vi "SeCrTs-Abort Executer.vi"(8 "error in":errorcluster, 11 "Message Queue":refnum<queue>) -> (0 "error IO":errorcluster)   [LabVIEW 2022 SP3]
uses:
  <vilib>/Platform/TimedLoop/XDataNode/timing_clust.ctl
  <vilib>/Platform/TimedLoop/XDataNode/nitl_modes.ctl
  <vilib>/Platform/TimedLoop/XDataNode/wakeup.ctl
  <vilib>/platform/TimedLoop/XDataNode/XDataNode.xnode
  <vilib>/Platform/TimedLoop/XDataNode/XDNodeRunTimeDep.lvlib
panel:
  out "Numeric":i32
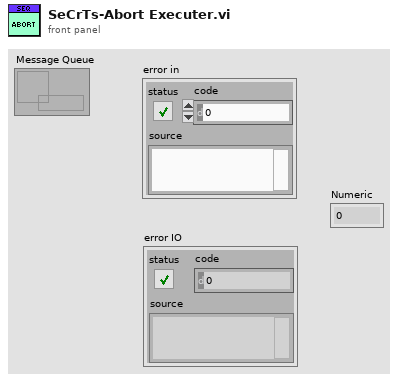
[diagram p1: front panel]
types:
  T1 = typedef "XDNodeRunTimeDep.lvlib/timing_clust.ctl" = cluster{"Expected End [f-1]":u64, "Actual End [f-1]":u64, "Finished Late? [f-1]":bool, "Expected End [i-1]":u64, "Actual End [i-1]":u64, "Finished Late? [i-1]":bool, "Expected Start [i]":u64, "Actual Start [i]":u64, "Expected Start [f]":u64, "Actual Start [f]":u64, "Source Name":string, "Structure Name":string, "Period":i64, "Deadline":i64, "Offset":i64, "Start":i64, "Priority":i32, "Timeout":i32, "Mode":T2, "Wakeup Reason":T3, "Error":errorcluster, "Source Type":string, "Secondary Source Type":string, "Global End Time":u64, "Global Start Time":u64, "Frame Duration":u64, "Iteration Duration":u64, "Assigned CPU":i32, "I/O Scan Engine Mode":u32}
  T2 = typedef "XDNodeRunTimeDep.lvlib/nitl_modes.ctl" = enum32{"No Change", "Process missed periods, maintain original phase", "Discard missed periods, maintain original phase", "Process missed periods, ignore original phase", "Discard missed periods, ignore original phase"}
  T3 = typedef "XDNodeRunTimeDep.lvlib/wakeup.ctl" = enum32{"Normal", "Aborted", "Asynchronous wakeup", "Timing source error", "Timed loop error", "Timeout"}
  T4 = enum16{"Init", "Read", "Write 'All'", "Write 'n'", "Write Safe Value", "Write Start Time", "Overwrite Pattern", "Overwrite Pattern with Start", "Append Pattern", "Start Pattern Mode", "Abort Pattern Mode", "Read 1"}
  T5 = cluster{"Start DAQ":bool, "Stop DAQ":bool, "RT Stop":bool, "RT Exit":bool, "Start Seq":bool}
  T6 = cluster{"Manual HOLD":bool, "Automatic Hold AI":bool, "Abort":bool, "Automatic Hold DI":bool}
  T7 = cluster{cluster{"Sr. No.":string, "Time CDT":string, "Component ID":string, "Data Type":string, "Condition":string, "Range/Position":string, "No of Samples for Pass":string, "Event Duration":string, "Continuous /Cumulative":string, "Expected Delay":string, "Failure case Seq":string, "Current Sequence":string}[]}[]
  T8 = cluster{"Sr. No.":string, "Time CDT":string, "Component ID":string, "Data Type":string, "Condition":string, "Range/Position":string, "No of Samples for Pass":string, "Event Duration":string, "Continuous /Cumulative":string, "Expected Delay":string, "Failure case Seq":string, "Current Sequence":string}[]
  T9 = cluster{"Sr. No.":string, "Time CDT":string, "Component ID":string, "Data Type":string, "Condition":string, "Range/Position":string, "No of Samples for Pass":string, "Event Duration":string, "Continuous /Cumulative":string, "Expected Delay":string, "Failure case Seq":string, "Current Sequence":string}
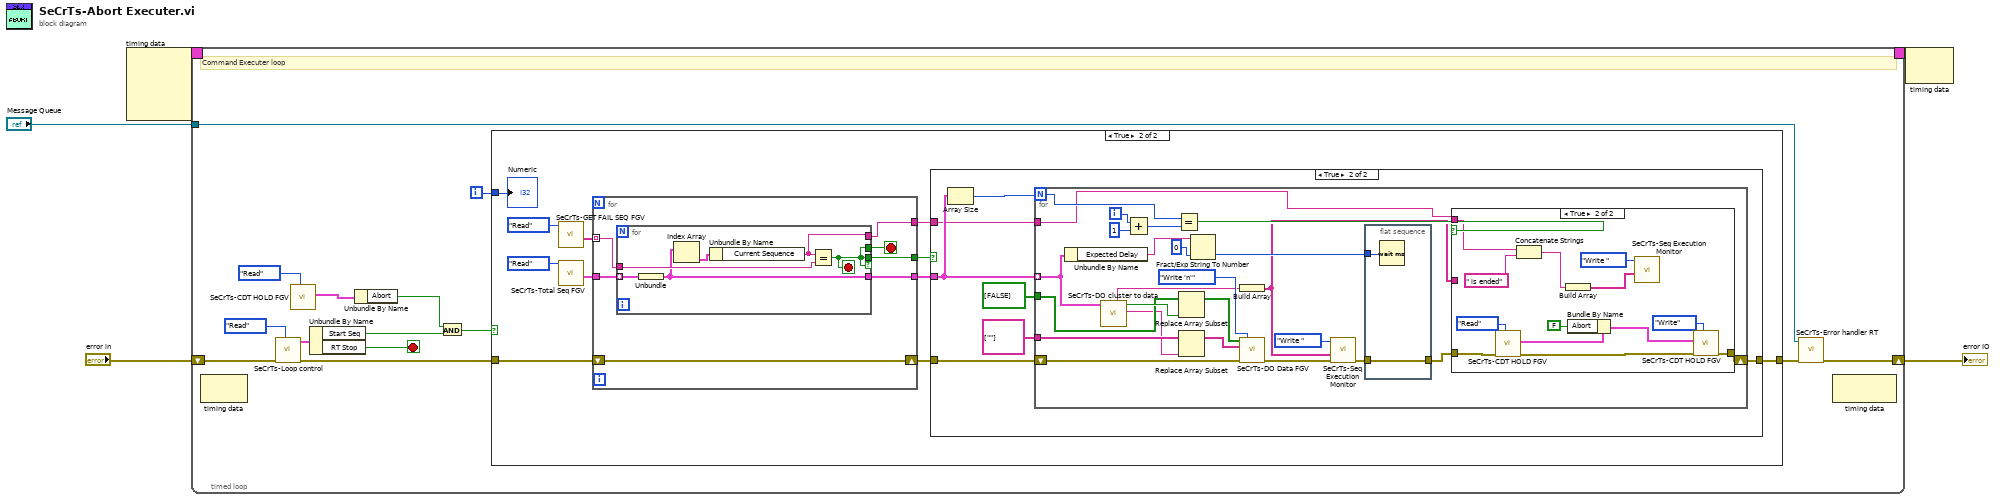
[diagram p0: block diagram]
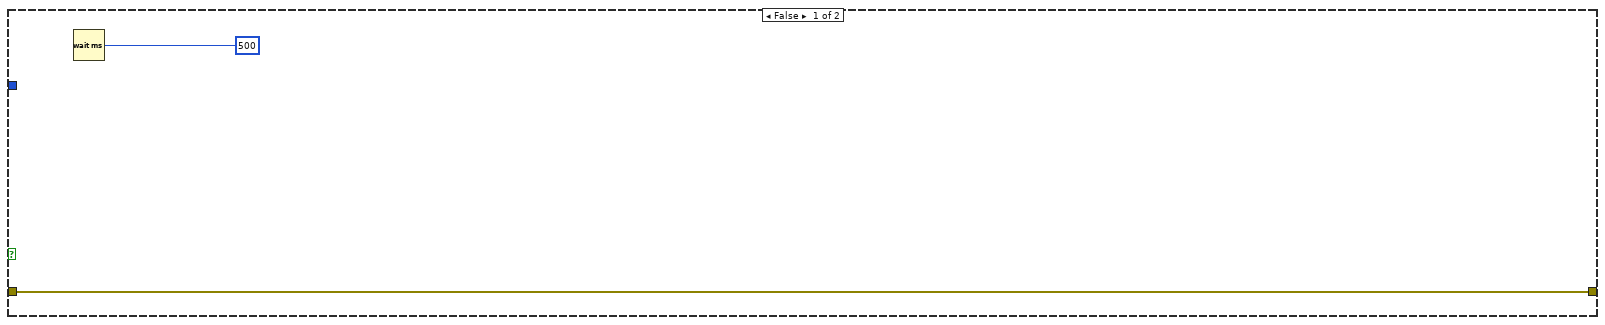
[diagram p2: hidden frame]
diagram:
  n1 = node-c288() -> (w3:T1)  [unwired: 4 in]
  n2 = timed-loop {
    shift-right: [w12] -> w4
    shift-left: "error in" -> [w17]
    timing: w3 -> [_]
    timing-out: [_] -> w2
    tunnel: "Message Queue" -> [w11]
    i -> [w18]
    stop <- w19 stop-if-true
    # "Command Executer loop"
    n3 = node-c288() -> ()  [unwired: 1 in, 1 out]
    n4 = call "SeCrTs-Loop control.vi"("Action"=enum16{"Init", "Write", "Read"}."Read", "error in (no error)"=w17) -> ("error Out"=w16:errorcluster, "Loop Control out"=w14:T5)  [unwired: 8 in]
    n5 = call "SeCrTs-CDT HOLD FGV.vi"("Write/Read"=enum16{"Write", "Read"}."Read") -> ("HOLD and Abort Out"=w8:T6)  [unwired: 7 in, 1 out]
    n6 = Unbundle By Name(w14) -> ("Start Seq"=w9:bool, "RT Stop"=w19:bool)
    n7 = Unbundle By Name(w8) -> ("Abort"=w6:bool)
    n8 = And(x=w6, y=w9) -> (x .and. y?=w7:bool)
    n9 = case shown="True" w7 {
      tunnel: [w21 w32] -> w13
      tunnel: w18 -> [_ w31]
      tunnel: w16 -> [w21 w24]
      frame False {
        n10 = Wait (ms)(milliseconds to wait=u32 500) -> ()  [unwired: 1 out]
      }
      frame True {
        n11 = call "SeCrTs-GET FAIL SEQ FGV.vi"("Enum"=enum16{"Read", "Write "}."Read") -> ("Failure \ncase Seq"=w25:string[])  [unwired: 9 in, 1 out]
        n12 = call "SeCrTs-Total Seq FGV.vi"("Enum"=enum16{"Read", "Write "}."Read") -> ("Total Seq  Out"=w28:T7)  [unwired: 9 in, 1 out]
        n13 = for {
          tunnel: [w35] -> w26
          tunnel: w28 -> [w36]
          tunnel: w25 -> [w39] mode=indexing
          tunnel: [w38] -> w27
          shift-right: [w34] -> w23
          shift-left: w24 -> [w34]
          tunnel: [w33] -> w22
          stop <- w37 stop-if-true
          n14 = for {
            tunnel: [w44] -> w38 if=w44
            tunnel: w39 -> [w45]
            tunnel: [w44] -> w37
            tunnel: w36 -> [w42] mode=indexing
            tunnel: [w41] -> w35
            tunnel: [w40] -> w33
            stop <- w44 stop-if-true
            n15 = Unbundle(w42) -> (w41:T8)
            n16 = Index Array(array=w41) -> (element=w43:T9)  [unwired: 1 in]
            n17 = Unbundle By Name(w43) -> ("Current Sequence"=w40:string)
            n18 = Equal?(x=w40, y=w45) -> (x = y?=w44:bool)
          }
        }
        n19 = case shown="True" w27 {
          tunnel: w23 -> [w46 w50]
          tunnel: [w46 w53] -> w32
          tunnel: w26 -> [_ w49]
          tunnel: w22 -> [_ w47]
          frame False {
          }
          frame True {
            n20 = Array Size(array=w49) -> (size(s)=w48:i32)
            n21 = for {
              N: w48 -> [w59]
              tunnel: w49 -> [w70] mode=indexing
              tunnel: string[] [""] ("appended array") -> [w78]
              tunnel: bool[] [FALSE] ("appended array") -> [w76]
              shift-right: [w56] -> w53
              shift-left: w50 -> [w71]
              tunnel: w47 -> [w55]
              i -> [w62]
              n22 = Unbundle By Name(w70) -> ("Expected Delay"=w73:string)
              n23 = call "SeCrTs-DO cluster to data.vi"("output cluster"=w70) -> ("Component ID"=w66:string, "Boolean"=w77:bool, "Sequence"=w63:string)  [unwired: 7 in, 1 out]
              n24 = Add(x=w62, y=1) -> (x+y=w60:i32)
              n25 = Equal?(x=w59, y=w60) -> (x = y?=w58:bool)
              n26 = Replace Array Subset(array=w76, new element=w77) -> (w75:bool[])  [unwired: 1 in]
              n27 = Replace Array Subset(array=w78, new element=w66) -> (w74:string[])  [unwired: 1 in]
              n28 = Fract/Exp String To Number(string=w73, default (0 dbl)=u32 0 ("y")) -> (number=w68:u32)  [unwired: 2 in, 1 out]
              n29 = Build Array(w63) -> (w54:string[])
              n30 = call "SeCrTs-DO Data FGV.vi"("DO Values In"=w75, "Option"=T4."Write 'n'", "DO Channel Names"=w74, "error in (no error)"=w71) -> ("error out"=w65:errorcluster)  [unwired: 5 in, 6 out]
              n31 = call "SeCrTs-Seq Execution Monitor.vi"("error in"=w65, "Seq Monitor"=w54, "Enum"=enum16{"Read", "Write "}."Write ") -> ("error out"=w64:errorcluster)  [unwired: 7 in, 1 out]
              n32 = flat-sequence {
                tunnel: w64 -> [w94]
                tunnel: [w94] -> w57
                tunnel: w68 -> [w93]
                frame #0 {
                  n33 = Wait (ms)(milliseconds to wait=w93) -> ()  [unwired: 1 out]
                }
              }
              n34 = case shown="True" w58 {
                tunnel: w57 -> [w79 w89]
                tunnel: [w79 w91] -> w56
                tunnel: w55 -> [_ w83]
                tunnel: w54 -> [_ _]
                frame False {
                }
                frame True {
                  n35 = call "SeCrTs-CDT HOLD FGV.vi"("Write/Read"=enum16{"Write", "Read"}."Read", "error in (no error)"=w89) -> ("error Out"=w88:errorcluster, "HOLD and Abort Out"=w87:T6)  [unwired: 6 in]
                  n36 = Concatenate Strings(w83, " is ended" ("string")) -> (w81:string)
                  n37 = Build Array(w81) -> (w80:string[])
                  n38 = Bundle By Name(cluster=w87, "Abort"=FALSE) -> (w85:T6)
                  n39 = call "SeCrTs-Seq Execution Monitor.vi"("Seq Monitor"=w80, "Enum"=enum16{"Read", "Write "}."Write ") -> ()  [unwired: 8 in, 2 out]
                  n40 = call "SeCrTs-CDT HOLD FGV.vi"("Write/Read"=enum16{"Write", "Read"}."Write", "error in (no error)"=w88, "HOLD and Abort"=w85) -> ("error Out"=w91:errorcluster)  [unwired: 5 in, 1 out]
                }
              }
            }
          }
        }
        "Numeric" <- w31
      }
    }
    n41 = call "SeCrTs-Error handler RT.vi"("error in"=w13, "Message Queue"=w11) -> ("error out"=w12:errorcluster)  [unwired: 8 in, 1 out]
    n42 = node-c288() -> ()  [unwired: 1 in, 1 out]
  }
  "error IO" <- w4
  n43 = node-c288(w2) -> ()  [unwired: 1 out]
